vi "delete module from engine.vi"(8 "error in":errorcluster, 10 "module ID":string, 11 "Standard Engine Configuration in":refnum<class "Standard Engine Configuration.lvclass">) -> (0 "error out":errorcluster, 3 "Standard Engine Configuration out":refnum<class "Standard Engine Configuration.lvclass">)   [LabVIEW 2013, in "Standard Engine Configuration.lvclass"]
uses:
  Standard Engine Configuration.lvclass
  Standard Engine Configuration.lvclass/Standard Engine Configuration.ctl
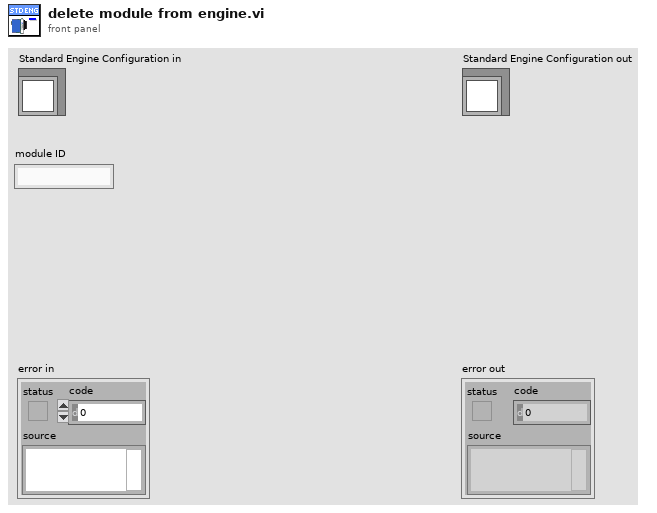
[diagram p1: front panel]
types:
  T1 = typedef "Standard Engine Configuration.lvclass/Module Specific Configuration.ctl" = cluster{"Module ID":string, "Module Decimation":T2, "Module Error Configuration":T3}
  T2 = typedef "Standard Engine Configuration.lvclass/Module Decimation.ctl" = cluster{"Decimation":u16, "Offset":u16}
  T3 = typedef "Standard Engine Configuration.lvclass/Module Error Configuration.ctl" = cluster{"Module Error Configuration":T4[]}
  T4 = typedef "Standard Engine Configuration.lvclass/Error Actions By Category.ctl" = cluster{"error classification":T5, "Error Actions":T6[]}
  T5 = typedef "TBM module execution interface.lvclass/error classification.ctl" = enum16{"unknown", "none", "trivial", "recoverable", "critical"}
  T6 = typedef "Standard Engine Configuration.lvclass/Error Actions.ctl" = enum16{"Clear", "Notify", "Stop Component", "Stop Engine", "Safe State", "Attempt Recovery"}
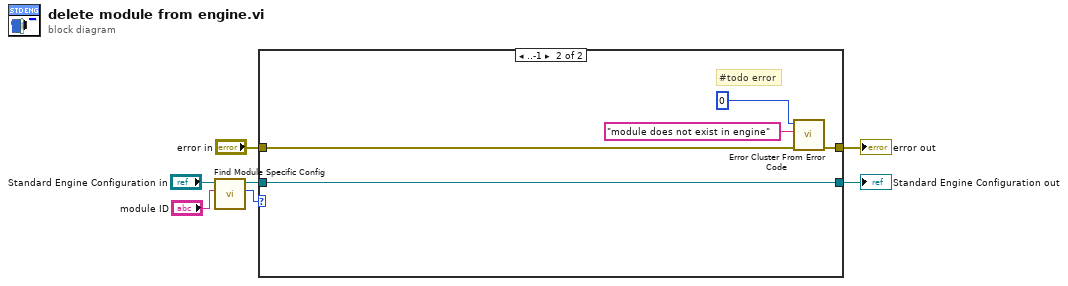
[diagram p0: block diagram]
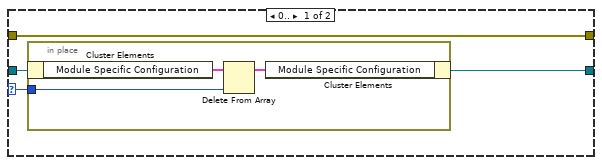
[diagram p2: hidden frame]
diagram:
  n1 = call "Find Module Specific Config.vi"("Module ID"="module ID", "Standard Engine Repo Data in"="Standard Engine Configuration in") -> ("Index"=w3:i32, "Standard Engine Repo Data out"=w5:refnum<class "Standard Engine Configuration.lvclass">)  [unwired: 8 in]
  n2 = case shown="..-1" w3 {
    selector: w3 -> [w8 _]
    tunnel: [w11 w19] -> w7
    tunnel: w5 -> [w10 w19]
    tunnel: "error in" -> [w9 w18]
    tunnel: [w9 w17] -> w2
    frame 0.. {
      n3 = in-place {
        in-place-border: w8 -> [w12]
        n4 = in-place-cluster #1(w10) -> ("Module Specific Configuration"=w14:T1[])
        n5 = Delete From Array(array=w14, index=w12) -> (array with subset deleted=w13:T1[])  [unwired: 1 in, 1 out]
        n6 = in-place-cluster #1("Module Specific Configuration"=w13) -> (w11:refnum<class "Standard Engine Configuration.lvclass">)
      }
    }
    frame ..-1 {
      # "#todo error"
      n7 = call <vilib>:"Error Cluster From Error Code.vi"("error in (no error)"=w18, "error message (\"\")"="module does not exist in engine" ("error message (\"\")"), "error code (0)"=0) -> ("error out"=w17:errorcluster)  [unwired: 6 in]
    }
  }
  "error out" <- w2
  "Standard Engine Configuration out" <- w7
